vi "autonSample.vi"(0 "Auton Array":dbl[][](array[numeric]), 5 "LeftEncoder":dbl, 7 "RightEncoder":dbl, 11 "MeasuredHeading":dbl) -> (4 "Left Drive":dbl, 6 "Right Drive":dbl, 8 "Ramp ACT motor":dbl, 10 "Harvester":dbl, 13 "Shooter motor output":dbl, 14 "Turret Rotation":dbl, 15 "Convyeor":dbl)   [LabVIEW 2011]
uses:
  <vilib>/addons/Kinect/Skeleton Vertex Index.ctl
  Robot Global Data.vi
panel:
  out "Primitive ID":i16
  out "Tzero":i64
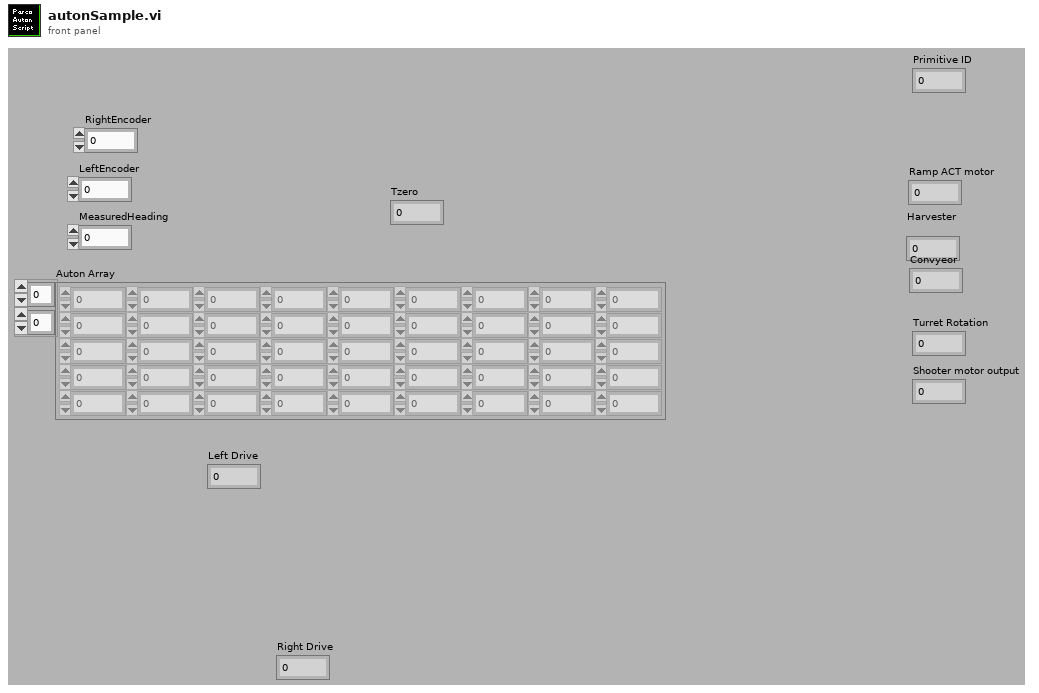
[diagram p1: front panel]
types:
  T1 = typedef "Skeleton Vertex Index.ctl" = i32
  T2 = cluster{"RightAxis":dbl, "LeftAxis":dbl, "RightHead":bool, "Left Head":bool, "Left Leg Out":bool, "Left Leg Forward":bool, "Left Leg Back":bool, "Right Leg Out":bool, "Right Leg Forward":bool, "Right Leg Back":bool}
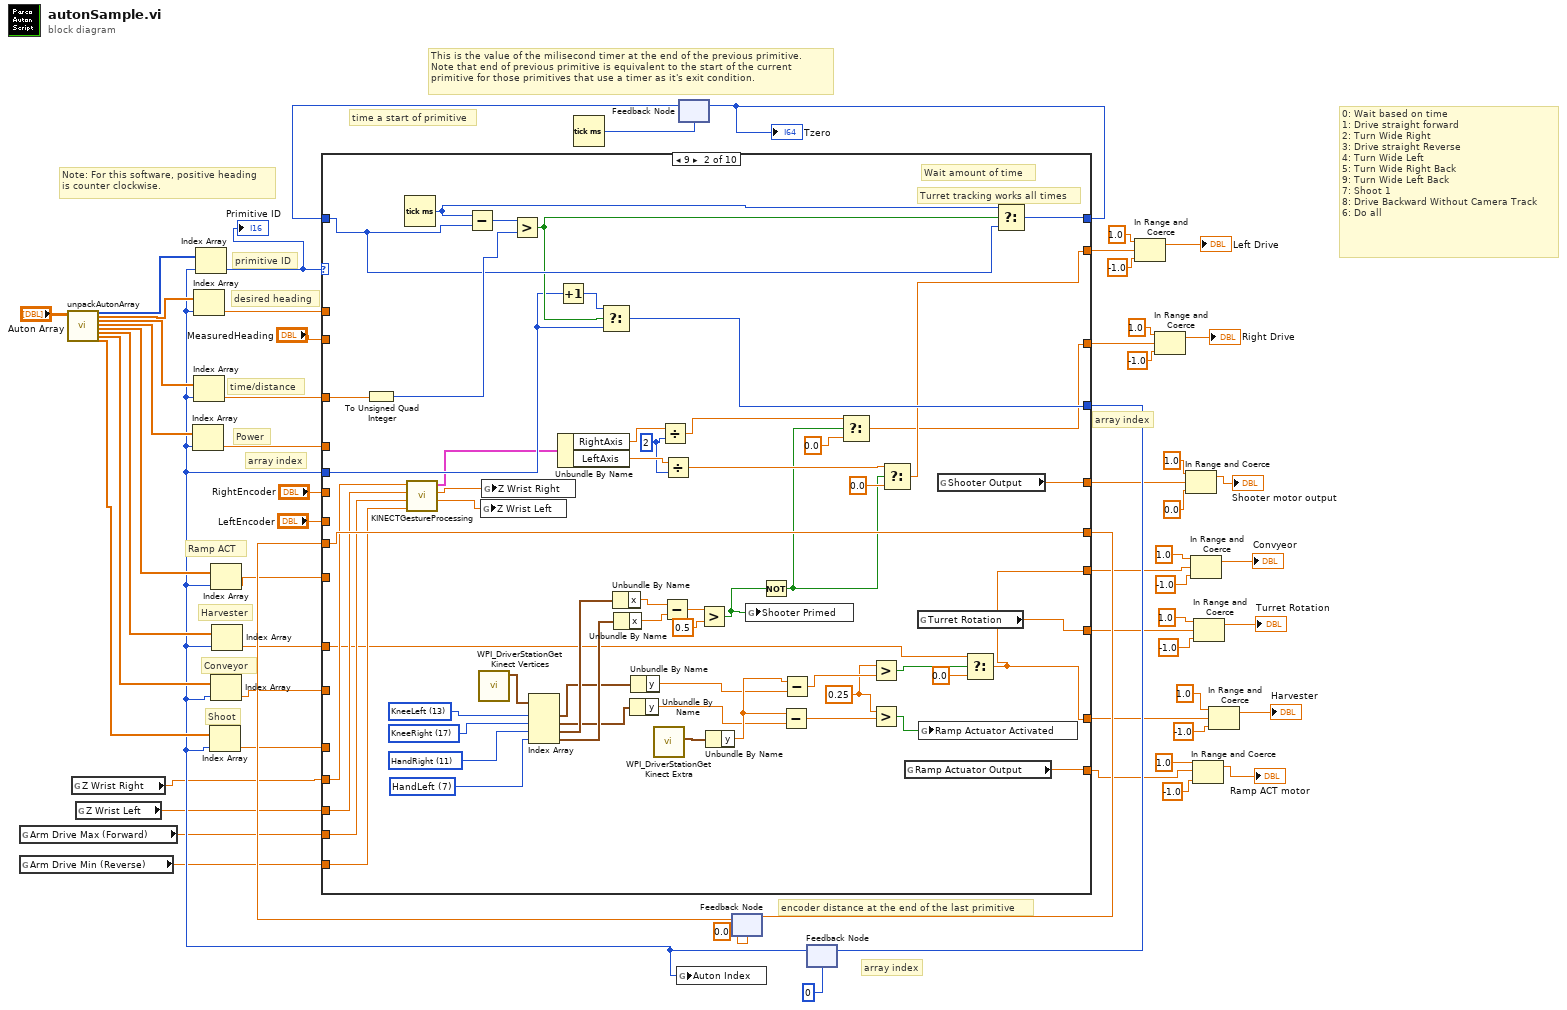
[diagram p0: block diagram]
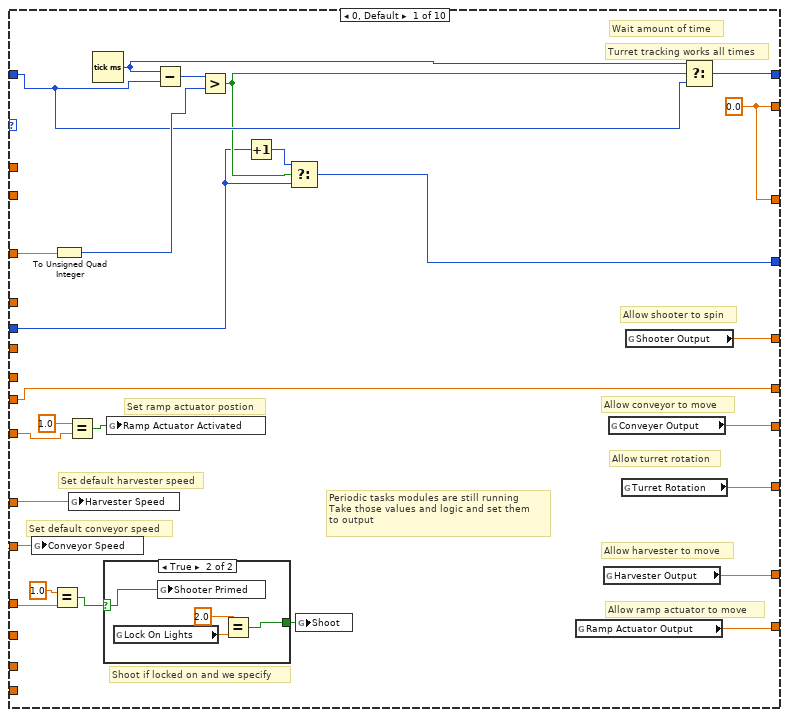
[diagram p2: hidden frame]
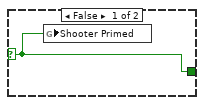
[diagram p3: hidden frame]
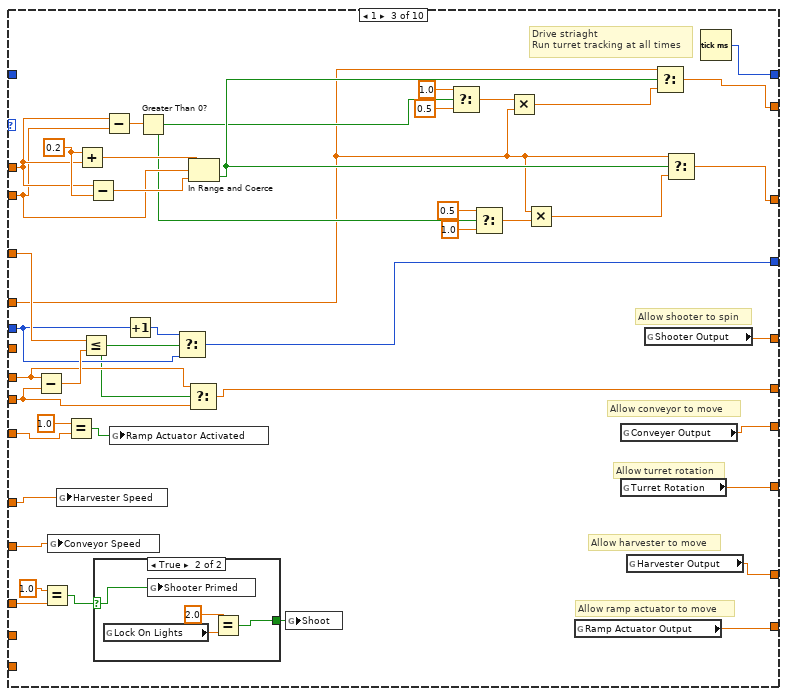
[diagram p4: hidden frame]
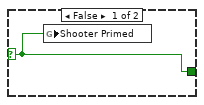
[diagram p5: hidden frame]
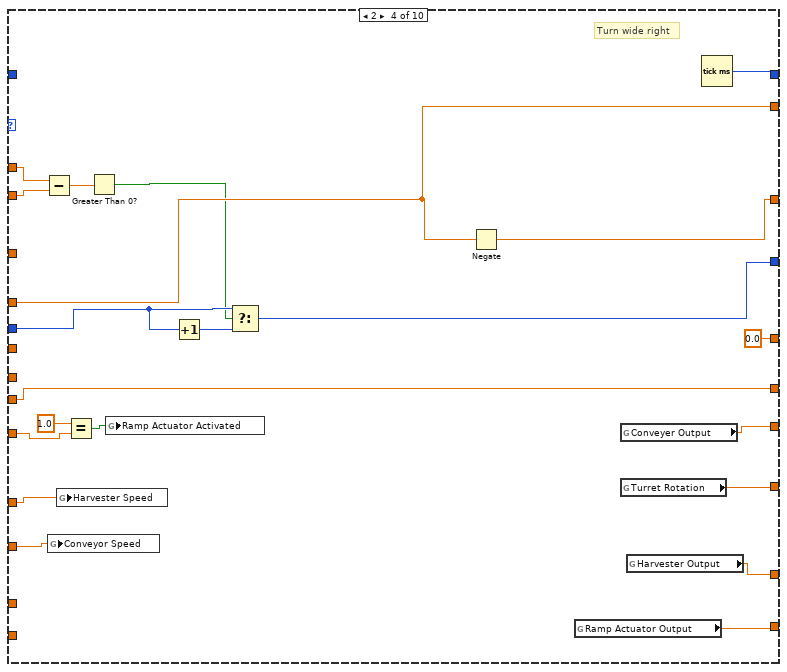
[diagram p6: hidden frame]
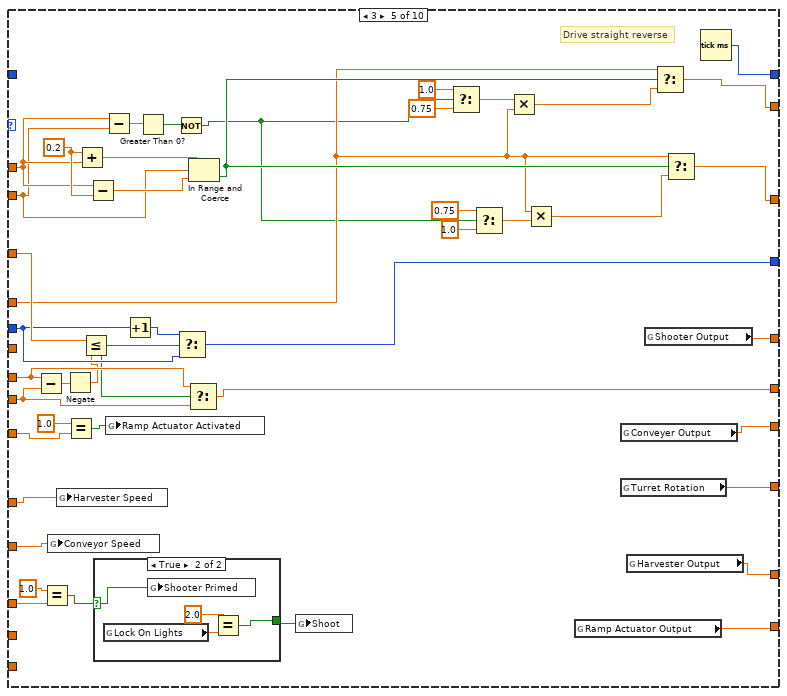
[diagram p7: hidden frame]
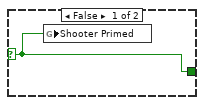
[diagram p8: hidden frame]
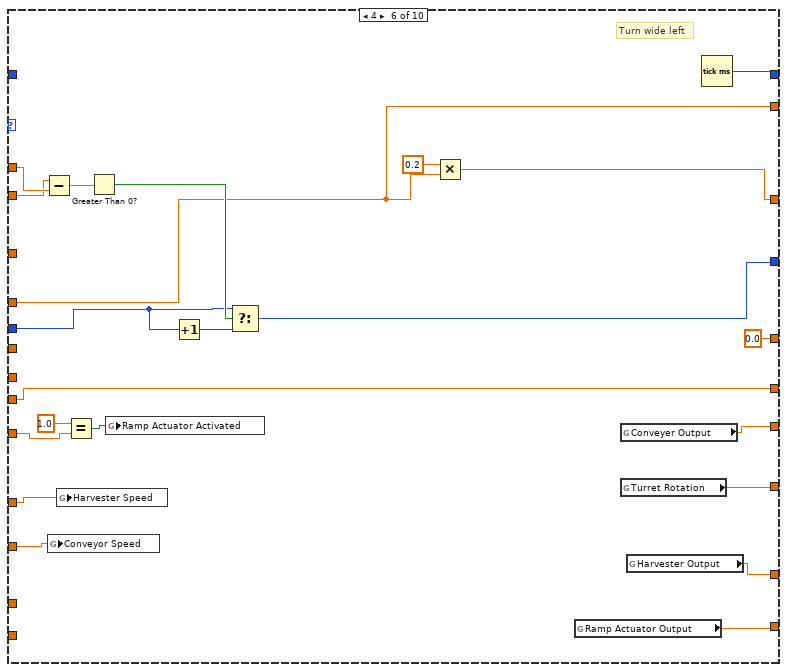
[diagram p9: hidden frame]
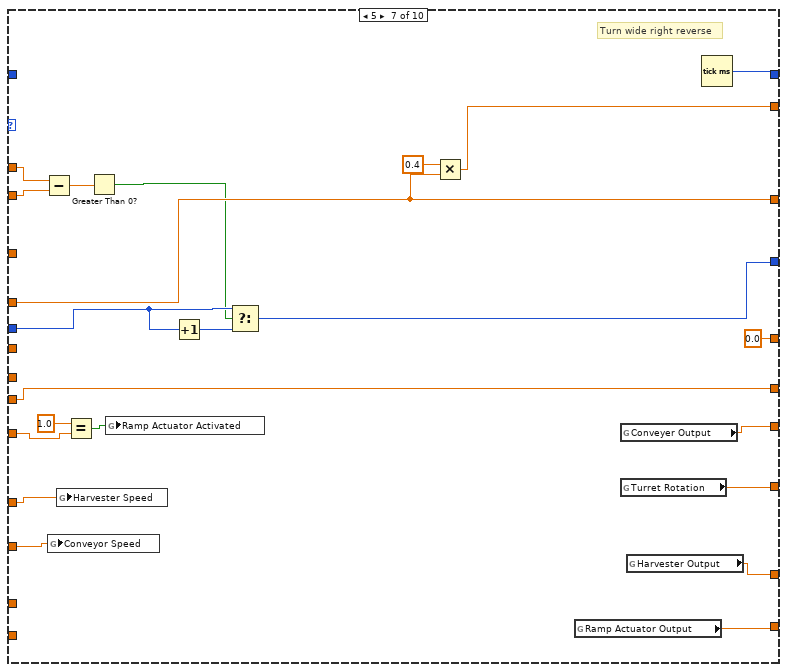
[diagram p10: hidden frame]
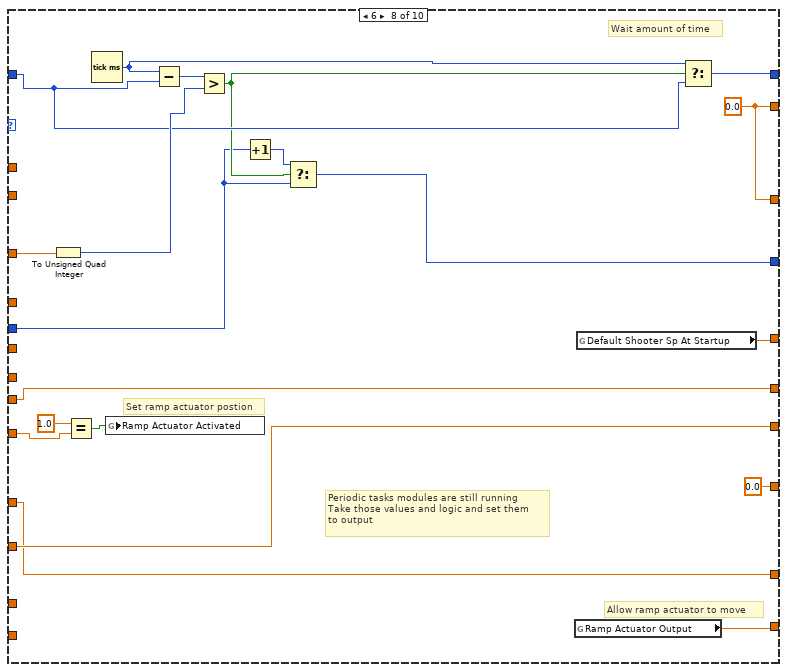
[diagram p11: hidden frame]
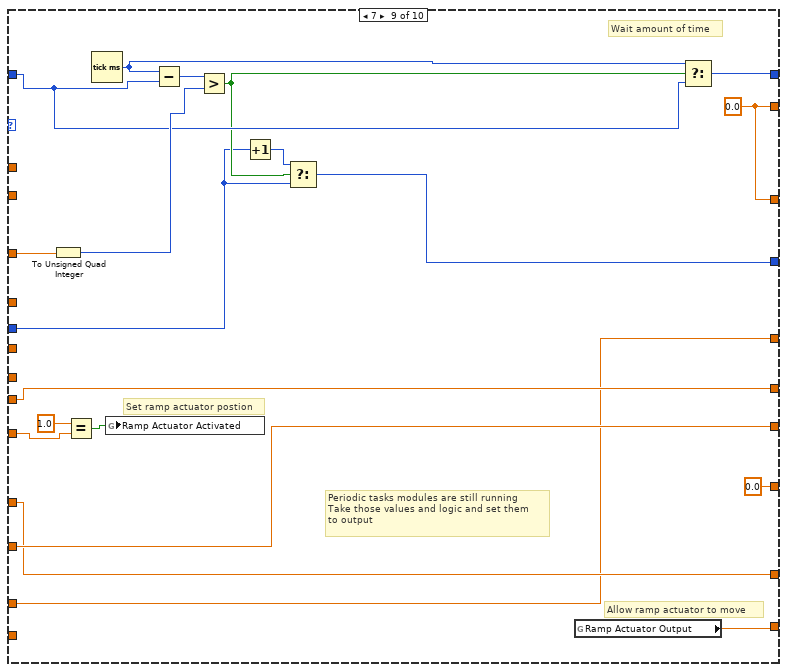
[diagram p12: hidden frame]
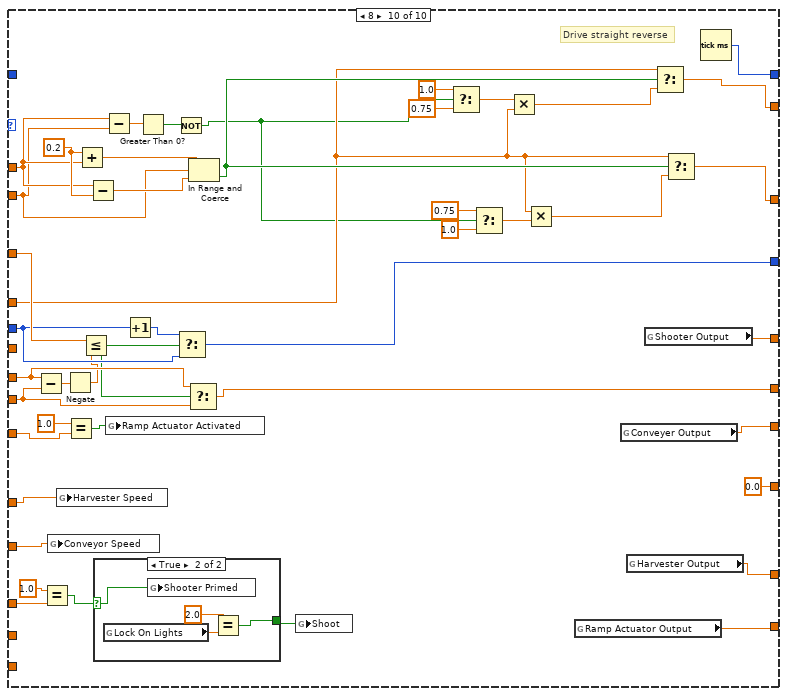
[diagram p13: hidden frame]
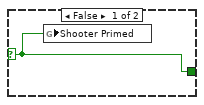
[diagram p14: hidden frame]
diagram:
  # "0: Wait based on time\n1: Drive straight forward\n2: Turn Wide Right\n3: Drive straight Reverse\n4: Turn Wide Left\n5: Turn Wide Right Back\n9: Turn Wide Left Back\n7: Shoot 1\n8: Drive Backward Without Camera Track\n6: Do all"
  # "Shoot"
  # "Conveyor"
  # "Harvester"
  # "Ramp ACT"
  # "encoder distance at the end of the last primitive"
  # "Note: For this software, positive heading\nis counter clockwise."
  # "time a start of primitive"
  # "array index"
  # "array index"
  # "This is the value of the milisecond timer at the end of the previous primitive.\nNote that end of previous primitive is equivalent to the start of the current\nprimitive for those primitives that use a timer as it's exit condition."
  # "Power"
  # "array index"
  # "desired heading"
  # "primitive ID"
  # "time/distance"
  n1 = global read "Robot Global Data.vi" "Arm Drive Max (Forward)"() -> (w2:dbl)
  n2 = global read "Robot Global Data.vi" "Arm Drive Min (Reverse)"() -> (w1:dbl)
  n3 = call "unpackAutonArray.vi"("all rows"="Auton Array") -> ("Primitive"=w60:i16[], "Desired Heading"=w20:dbl[], "Time/Distance"=w19:dbl[], "Power"=w18:dbl[], "Ramp Actuator"=w17:dbl[], "Harvester"=w16:dbl[], "Conveyor"=w15:dbl[], "Shoot"=w14:dbl[])  [unwired: 1 in, 18 out]
  n4 = global read "Robot Global Data.vi" "Z Wrist Right"() -> (w4:dbl)
  n5 = global read "Robot Global Data.vi" "Z Wrist Left"() -> (w3:dbl)
  n6 = Tick Count (ms)() -> (millisecond timer value=w55:u32)
  n7 = feedback #1(w55) -> (w59:u32)
  n8 = feedback #2(0.0 ("EncoderDistance")) -> (w43:dbl)
  n9 = feedback #3(0) -> (w12:i32)
  n10 = Index Array(array=w18, index=w12) -> (element=w57:dbl)
  n11 = Index Array(array=w20, index=w12) -> (element=w44:dbl)
  n12 = Index Array(array=w19, index=w12) -> (element=w58:dbl)
  n13 = Index Array(array=w60, index=w12) -> (element=w26:i16)
  "Primitive ID" <- w26
  n14 = Index Array(array=w14, index=w12) -> (element=w13:dbl)
  n15 = Index Array(array=w17, index=w12) -> (element=w25:dbl)
  n16 = Index Array(array=w15, index=w12) -> (element=w10:dbl)
  n17 = Index Array(array=w16, index=w12) -> (element=w11:dbl)
  n18 = case shown="9" w26 {
    tunnel: [w79 w141 w175 w201 w247 w274 w292 w324 w344 w382] -> w39
    tunnel: w12 -> [w80 w142 w177 w203 w249 w276 w294 w325 w345 w384]
    tunnel: [w87 w149 w153 w207 w226 w280 w301 w332 w352 w361] -> w45
    tunnel: w59 -> [w84 w146 _ _ _ _ _ w329 w349 _]
    tunnel: w58 -> [w73 w140 w178 _ w250 _ _ w319 w339 w385]
    tunnel: w44 -> [_ _ w166 w206 w238 w271 w300 _ _ w373]
    tunnel: [w78 w123 w152 w200 w225 w273 w296 w323 w343 w360] -> w53
    tunnel: [w78 w122 w151 w199 w224 w272 w298 w323 w343 w359] -> w46
    tunnel: w57 -> [_ _ w155 w200 w228 w273 w298 _ _ w363]
    tunnel: "LeftEncoder" -> [_ _ w172 _ w244 _ _ _ _ w379]
    tunnel: "MeasuredHeading" -> [_ _ w165 w205 w237 w270 w299 _ _ w372]
    tunnel: [w72 w139 w174 w209 w246 w282 w303 w318 w338 w381] -> w40
    tunnel: w43 -> [w72 w139 w173 w209 w245 w282 w303 w318 w338 w380]
    tunnel: [w62 w138 w180 0.0 ("Shooter Output") w251 0.0 ("Shooter Output") 0.0 ("Shooter Output") w313 w333 w386] -> w35
    tunnel: [w74 w95 w190 w215 w260 w287 w309 0.0 ("Turret Rotation") 0.0 ("Turret Rotation") 0.0 ("Turret Rotation")] -> w31
    tunnel: [w70 w96 w184 w211 w255 w284 w305 w315 w335 w390] -> w27
    tunnel: w25 -> [w67 _ w187 w214 w223 w269 w308 w317 w337 w358]
    tunnel: [w75 w94 w191 w216 w261 w288 w310 w320 w340 w395] -> w24
    tunnel: w13 -> [w63 _ w188 _ w258 _ _ _ w333 w393]
    tunnel: w11 -> [w68 w97 w186 w213 w257 w286 w307 w315 w335 w392]
    tunnel: w10 -> [w69 _ w185 w212 w256 w285 w306 w316 w336 w391]
    tunnel: [w71 w96 w183 w210 w254 w283 w304 w316 w336 w389] -> w6
    tunnel: "RightEncoder" -> [_ _ _ _ _ _ _ _ _ _]
    tunnel: w4 -> [_ w137 _ _ _ _ _ _ _ _]
    tunnel: w3 -> [_ w136 _ _ _ _ _ _ _ _]
    tunnel: w2 -> [_ w135 _ _ _ _ _ _ _ _]
    tunnel: w1 -> [_ w134 _ _ _ _ _ _ _ _]
    frame 0, Default {
      w78 = 0.0 ("Numeric")
      # "Periodic tasks modules are still running\nTake those values and logic and set them \nto output"
      # "Set ramp actuator postion"
      # "Set default harvester speed"
      # "Set default conveyor speed"
      # "Shoot if locked on and we specify"
      # "Allow ramp actuator to move"
      # "Allow harvester to move"
      # "Turret tracking works all times"
      # "Allow turret rotation"
      # "Allow conveyor to move"
      # "Allow shooter to spin"
      # "Wait amount of time"
      n19 = global write "Robot Global Data.vi" "Conveyor Speed"(w69) -> ()
      n20 = Equal?(x=1.0, y=w63) -> (x = y?=w65:bool)
      n21 = To Unsigned Quad Integer(1:w73) -> (0:w85:u64)
      n22 = Equal?(x=1.0, y=w67) -> (x = y?=w76:bool)
      n23 = global write "Robot Global Data.vi" "Harvester Speed"(w68) -> ()
      n24 = Tick Count (ms)() -> (millisecond timer value=w83:u32)
      n25 = case shown="True" w65 {
        selector: w65 -> [w88 w92]
        tunnel: [w88 w89] -> w64
        frame False {
          n26 = global write "Robot Global Data.vi" "Shooter Primed"(w88) -> ()
        }
        frame True {
          n27 = global read "Robot Global Data.vi" "Lock On Lights"() -> (w90:dbl)
          n28 = global write "Robot Global Data.vi" "Shooter Primed"(w92) -> ()
          n29 = Equal?(x=2.0, y=w90) -> (x = y?=w89:bool)
        }
      }
      n30 = global write "Robot Global Data.vi" "Ramp Actuator Activated"(w76) -> ()
      n31 = Subtract(x=w83, y=w84) -> (x-y=w86:u32)
      n32 = Greater?(x=w86, y=w85) -> (0:w82:bool)
      n33 = Increment(x=w80) -> (x+1=w81:i32)
      n34 = Select(t=w81, s=w82, f=w80) -> (s? t:f=w79:i32)
      n35 = global write "Robot Global Data.vi" "Shoot"(w64) -> ()
      n36 = global read "Robot Global Data.vi" "Ramp Actuator Output"() -> (w75:dbl)
      n37 = global read "Robot Global Data.vi" "Harvester Output"() -> (w70:dbl)
      n38 = global read "Robot Global Data.vi" "Conveyer Output"() -> (w71:dbl)
      n39 = global read "Robot Global Data.vi" "Turret Rotation"() -> (w74:dbl)
      n40 = global read "Robot Global Data.vi" "Shooter Output"() -> (w62:dbl)
      n41 = Select(t=w83, s=w82, f=w84) -> (s? t:f=w87:u32)
    }
    frame 9 {
      w100 = 0.25
      w117 = T1 7 items=["HipCenter", "Spine", "ShoulderCenter", "Head", "ShoulderLeft", "ElbowLeft", "WristLeft", "HandLeft", "ShoulderRight", "ElbowRight", "WristRight", "HandRight", "HipLeft", "KneeLeft", "AnkleLeft", "FootLeft", "HipRight", "KneeRight", "AnkleRight", "FootRight"] ("Skeleton Joints")
      w118 = T1 11 items=["HipCenter", "Spine", "ShoulderCenter", "Head", "ShoulderLeft", "ElbowLeft", "WristLeft", "HandLeft", "ShoulderRight", "ElbowRight", "WristRight", "HandRight", "HipLeft", "KneeLeft", "AnkleLeft", "FootLeft", "HipRight", "KneeRight", "AnkleRight", "FootRight"] ("Skeleton Joints")
      w119 = T1 17 items=["HipCenter", "Spine", "ShoulderCenter", "Head", "ShoulderLeft", "ElbowLeft", "WristLeft", "HandLeft", "ShoulderRight", "ElbowRight", "WristRight", "HandRight", "HipLeft", "KneeLeft", "AnkleLeft", "FootLeft", "HipRight", "KneeRight", "AnkleRight", "FootRight"] ("Skeleton Joints")
      w120 = T1 13 items=["HipCenter", "Spine", "ShoulderCenter", "Head", "ShoulderLeft", "ElbowLeft", "WristLeft", "HandLeft", "ShoulderRight", "ElbowRight", "WristRight", "HandRight", "HipLeft", "KneeLeft", "AnkleLeft", "FootLeft", "HipRight", "KneeRight", "AnkleRight", "FootRight"] ("Skeleton Joints")
      w128 = 2
      # "Turret tracking works all times"
      # "Wait amount of time"
      n42 = To Unsigned Quad Integer(1:w140) -> (0:w147:u64)
      n43 = Tick Count (ms)() -> (millisecond timer value=w145:u32)
      n44 = call "KINECTGestureProcessing.vi"("Z Wrist Right in"=w137, "Z Wrist Left in"=w136, "Arm Drive in Max (Forward)"=w135, "Arm Drive in Min (Reverse)"=w134) -> ("Joystick Data"=w131:T2, "Z Wrist Right out"=w133:dbl, "Z Wrist Left out"=w132:dbl)  [unwired: 2 in]
      n45 = Subtract(x=w145, y=w146) -> (x-y=w148:u32)
      n46 = call <vilib>:"WPI_DriverStationGet Kinect Vertices.vi"() -> ("Skeleton Vertices"=w121:cluster{"x":sgl, "y":sgl, "z":sgl}[])  [unwired: 10 in, 1 out]
      n47 = global write "Robot Global Data.vi" "Z Wrist Left"(w132) -> ()
      n48 = global write "Robot Global Data.vi" "Z Wrist Right"(w133) -> ()
      n49 = Greater?(x=w148, y=w147) -> (0:w144:bool)
      n50 = Index Array(array=w121, index #1=w120, index #2=w119, index #3=w118, index #4=w117) -> (element #1=w114:cluster{"x":sgl, "y":sgl, "z":sgl}, element #2=w113:cluster{"x":sgl, "y":sgl, "z":sgl}, element #3=w116:cluster{"x":sgl, "y":sgl, "z":sgl}, element #4=w115:cluster{"x":sgl, "y":sgl, "z":sgl})
      n51 = Increment(x=w142) -> (x+1=w143:i32)
      n52 = Unbundle By Name(w131) -> ("RightAxis"=w130:dbl, "LeftAxis"=w129:dbl)
      n53 = Select(t=w143, s=w144, f=w142) -> (s? t:f=w141:i32)
      n54 = Unbundle By Name(w116) -> ("x"=w112:sgl)
      n55 = Unbundle By Name(w115) -> ("x"=w111:sgl)
      n56 = Unbundle By Name(w113) -> ("y"=w104:sgl)
      n57 = Unbundle By Name(w114) -> ("y"=w103:sgl)
      n58 = call <vilib>:"WPI_DriverStationGet Kinect Extra.vi"() -> ("Overall Position"=w106:cluster{"x":sgl, "y":sgl, "z":sgl})  [unwired: 7 in, 4 out]
      n59 = Divide(x=w130, y=w128) -> (x/y=w127:dbl)
      n60 = Subtract(x=w112, y=w111) -> (x-y=w110:sgl)
      n61 = Divide(x=w129, y=w128) -> (x/y=w126:dbl)
      n62 = Greater?(x=w110, y=sgl 0.5) -> (0:w108:bool)
      n63 = Unbundle By Name(w106) -> ("y"=w105:sgl)
      n64 = global write "Robot Global Data.vi" "Shooter Primed"(w108) -> ()
      n65 = Not(x=w108) -> (.not. x?=w107:bool)
      n66 = Subtract(x=w105, y=w104) -> (x-y=w102:sgl)
      n67 = Subtract(x=w105, y=w103) -> (x-y=w101:sgl)
      n68 = Select(t=w127, s=w107, f=0.0) -> (s? t:f=w122:dbl)
      n69 = Greater?(x=w100, y=w101) -> (0:w99:bool)
      n70 = Greater?(x=w100, y=w102) -> (0:w93:bool)
      n71 = Select(t=w126, s=w107, f=0.0) -> (s? t:f=w123:dbl)
      n72 = global read "Robot Global Data.vi" "Ramp Actuator Output"() -> (w94:dbl)
      n73 = global read "Robot Global Data.vi" "Turret Rotation"() -> (w95:dbl)
      n74 = global write "Robot Global Data.vi" "Ramp Actuator Activated"(w93) -> ()
      n75 = global read "Robot Global Data.vi" "Shooter Output"() -> (w138:dbl)
      n76 = Select(t=w97, s=w99, f=0.0) -> (s? t:f=w96:dbl)
      n77 = Select(t=w145, s=w144, f=w146) -> (s? t:f=w149:u32)
    }
    frame 1 {
      w170 = 0.2 ("x")
      # "Allow ramp actuator to move"
      # "Allow harvester to move"
      # "Allow turret rotation"
      # "Allow conveyor to move"
      # "Allow shooter to spin"
      # "Drive striaght\nRun turret tracking at all times"
      n78 = Subtract(x=w172, y=w173) -> (x-y=w179:dbl)
      n79 = Equal?(x=1.0, y=w188) -> (x = y?=w182:bool)
      n80 = global write "Robot Global Data.vi" "Conveyor Speed"(w185) -> ()
      n81 = global write "Robot Global Data.vi" "Harvester Speed"(w186) -> ()
      n82 = Equal?(x=1.0, y=w187) -> (x = y?=w150:bool)
      n83 = Add(x=w170, y=w166) -> (x+y=w168:dbl)
      n84 = Less Or Equal?(x=w178, y=w179) -> (x <= y?=w171:bool)
      n85 = Subtract(x=w166, y=w170) -> (x-y=w169:dbl)
      n86 = case shown="True" w182 {
        selector: w182 -> [w193 w197]
        tunnel: [w193 w194] -> w181
        frame False {
          n87 = global write "Robot Global Data.vi" "Shooter Primed"(w193) -> ()
        }
        frame True {
          n88 = global read "Robot Global Data.vi" "Lock On Lights"() -> (w195:dbl)
          n89 = global write "Robot Global Data.vi" "Shooter Primed"(w197) -> ()
          n90 = Equal?(x=2.0, y=w195) -> (x = y?=w194:bool)
        }
      }
      n91 = Subtract(x=w166, y=w165) -> (x-y=w164:dbl)
      n92 = global write "Robot Global Data.vi" "Ramp Actuator Activated"(w150) -> ()
      n93 = Increment(x=w177) -> (x+1=w176:i32)
      n94 = Greater Than 0?(x=w164) -> (x > 0?=w163:bool)
      n95 = Select(t=w176, s=w171, f=w177) -> (s? t:f=w175:i32)
      n96 = Select(t=w172, s=w171, f=w173) -> (s? t:f=w174:dbl)
      n97 = In Range and Coerce(upper limit=w168, x=w165, lower limit=w169) -> (In Range?=w167:bool)  [unwired: 1 out]
      n98 = global write "Robot Global Data.vi" "Shoot"(w181) -> ()
      n99 = Select(t=1.0, s=w163, f=0.5) -> (s? t:f=w156:dbl)
      n100 = Select(t=0.5, s=w163, f=1.0) -> (s? t:f=w158:dbl)
      n101 = Multiply(x=w156, y=w155) -> (x*y=w154:dbl)
      n102 = Multiply(x=w155, y=w158) -> (x*y=w157:dbl)
      n103 = global read "Robot Global Data.vi" "Ramp Actuator Output"() -> (w191:dbl)
      n104 = global read "Robot Global Data.vi" "Conveyer Output"() -> (w183:dbl)
      n105 = global read "Robot Global Data.vi" "Turret Rotation"() -> (w190:dbl)
      n106 = global read "Robot Global Data.vi" "Harvester Output"() -> (w184:dbl)
      n107 = global read "Robot Global Data.vi" "Shooter Output"() -> (w180:dbl)
      n108 = Select(t=w155, s=w167, f=w154) -> (s? t:f=w152:dbl)
      n109 = Select(t=w155, s=w167, f=w157) -> (s? t:f=w151:dbl)
      n110 = Tick Count (ms)() -> (millisecond timer value=w153:u32)
    }
    frame 2 {
      # "Turn wide right"
      n111 = Subtract(x=w206, y=w205) -> (x-y=w204:dbl)
      n112 = global write "Robot Global Data.vi" "Conveyor Speed"(w212) -> ()
      n113 = global write "Robot Global Data.vi" "Harvester Speed"(w213) -> ()
      n114 = Equal?(x=1.0, y=w214) -> (x = y?=w217:bool)
      n115 = Greater Than 0?(x=w204) -> (x > 0?=w198:bool)
      n116 = global write "Robot Global Data.vi" "Ramp Actuator Activated"(w217) -> ()
      n117 = Increment(x=w203) -> (x+1=w202:i32)
      n118 = Select(t=w203, s=w198, f=w202) -> (s? t:f=w201:i32)
      n119 = Negate(x=w200) -> (-x=w199:dbl)
      n120 = global read "Robot Global Data.vi" "Ramp Actuator Output"() -> (w216:dbl)
      n121 = global read "Robot Global Data.vi" "Conveyer Output"() -> (w210:dbl)
      n122 = global read "Robot Global Data.vi" "Turret Rotation"() -> (w215:dbl)
      n123 = global read "Robot Global Data.vi" "Harvester Output"() -> (w211:dbl)
      n124 = Tick Count (ms)() -> (millisecond timer value=w207:u32)
    }
    frame 3 {
      w242 = 0.2 ("x")
      # "Drive straight reverse"
      n125 = Subtract(x=w244, y=w245) -> (x-y=w222:dbl)
      n126 = Equal?(x=1.0, y=w258) -> (x = y?=w253:bool)
      n127 = global write "Robot Global Data.vi" "Conveyor Speed"(w256) -> ()
      n128 = global write "Robot Global Data.vi" "Harvester Speed"(w257) -> ()
      n129 = Negate(x=w222) -> (-x=w221:dbl)
      n130 = Equal?(x=1.0, y=w223) -> (x = y?=w262:bool)
      n131 = Add(x=w242, y=w238) -> (x+y=w240:dbl)
      n132 = Less Or Equal?(x=w250, y=w221) -> (x <= y?=w243:bool)
      n133 = Subtract(x=w238, y=w242) -> (x-y=w241:dbl)
      n134 = case shown="True" w253 {
        selector: w253 -> [w264 w268]
        tunnel: [w264 w265] -> w252
        frame False {
          n135 = global write "Robot Global Data.vi" "Shooter Primed"(w264) -> ()
        }
        frame True {
          n136 = global read "Robot Global Data.vi" "Lock On Lights"() -> (w266:dbl)
          n137 = global write "Robot Global Data.vi" "Shooter Primed"(w268) -> ()
          n138 = Equal?(x=2.0, y=w266) -> (x = y?=w265:bool)
        }
      }
      n139 = Subtract(x=w238, y=w237) -> (x-y=w236:dbl)
      n140 = global write "Robot Global Data.vi" "Ramp Actuator Activated"(w262) -> ()
      n141 = Increment(x=w249) -> (x+1=w248:i32)
      n142 = Greater Than 0?(x=w236) -> (x > 0?=w220:bool)
      n143 = Not(x=w220) -> (.not. x?=w219:bool)
      n144 = Select(t=w248, s=w243, f=w249) -> (s? t:f=w247:i32)
      n145 = Select(t=w244, s=w243, f=w245) -> (s? t:f=w246:dbl)
      n146 = In Range and Coerce(upper limit=w240, x=w237, lower limit=w241) -> (In Range?=w239:bool)  [unwired: 1 out]
      n147 = global write "Robot Global Data.vi" "Shoot"(w252) -> ()
      n148 = Select(t=1.0, s=w219, f=0.75) -> (s? t:f=w229:dbl)
      n149 = Select(t=0.75, s=w219, f=1.0) -> (s? t:f=w231:dbl)
      n150 = Multiply(x=w229, y=w228) -> (x*y=w227:dbl)
      n151 = Multiply(x=w228, y=w231) -> (x*y=w230:dbl)
      n152 = global read "Robot Global Data.vi" "Ramp Actuator Output"() -> (w261:dbl)
      n153 = global read "Robot Global Data.vi" "Conveyer Output"() -> (w254:dbl)
      n154 = global read "Robot Global Data.vi" "Turret Rotation"() -> (w260:dbl)
      n155 = global read "Robot Global Data.vi" "Harvester Output"() -> (w255:dbl)
      n156 = global read "Robot Global Data.vi" "Shooter Output"() -> (w251:dbl)
      n157 = Select(t=w228, s=w239, f=w227) -> (s? t:f=w225:dbl)
      n158 = Select(t=w228, s=w239, f=w230) -> (s? t:f=w224:dbl)
      n159 = Tick Count (ms)() -> (millisecond timer value=w226:u32)
    }
    frame 4 {
      # "Turn wide left"
      n160 = Subtract(x=w270, y=w271) -> (x-y=w278:dbl)
      n161 = global write "Robot Global Data.vi" "Conveyor Speed"(w285) -> ()
      n162 = global write "Robot Global Data.vi" "Harvester Speed"(w286) -> ()
      n163 = Equal?(x=1.0, y=w269) -> (x = y?=w289:bool)
      n164 = Greater Than 0?(x=w278) -> (x > 0?=w277:bool)
      n165 = global write "Robot Global Data.vi" "Ramp Actuator Activated"(w289) -> ()
      n166 = Increment(x=w276) -> (x+1=w275:i32)
      n167 = Select(t=w276, s=w277, f=w275) -> (s? t:f=w274:i32)
      n168 = Multiply(x=0.2, y=w273) -> (x*y=w272:dbl)
      n169 = global read "Robot Global Data.vi" "Ramp Actuator Output"() -> (w288:dbl)
      n170 = global read "Robot Global Data.vi" "Conveyer Output"() -> (w283:dbl)
      n171 = global read "Robot Global Data.vi" "Turret Rotation"() -> (w287:dbl)
      n172 = global read "Robot Global Data.vi" "Harvester Output"() -> (w284:dbl)
      n173 = Tick Count (ms)() -> (millisecond timer value=w280:u32)
    }
    frame 5 {
      # "Turn wide right reverse"
      n174 = Subtract(x=w300, y=w299) -> (x-y=w295:dbl)
      n175 = global write "Robot Global Data.vi" "Conveyor Speed"(w306) -> ()
      n176 = global write "Robot Global Data.vi" "Harvester Speed"(w307) -> ()
      n177 = Equal?(x=1.0, y=w308) -> (x = y?=w311:bool)
      n178 = Greater Than 0?(x=w295) -> (x > 0?=w291:bool)
      n179 = global write "Robot Global Data.vi" "Ramp Actuator Activated"(w311) -> ()
      n180 = Increment(x=w294) -> (x+1=w293:i32)
      n181 = Select(t=w294, s=w291, f=w293) -> (s? t:f=w292:i32)
      n182 = Multiply(x=0.4, y=w298) -> (x*y=w296:dbl)
      n183 = global read "Robot Global Data.vi" "Ramp Actuator Output"() -> (w310:dbl)
      n184 = global read "Robot Global Data.vi" "Conveyer Output"() -> (w304:dbl)
      n185 = global read "Robot Global Data.vi" "Turret Rotation"() -> (w309:dbl)
      n186 = global read "Robot Global Data.vi" "Harvester Output"() -> (w305:dbl)
      n187 = Tick Count (ms)() -> (millisecond timer value=w301:u32)
    }
    frame 6 {
      w323 = 0.0 ("Numeric")
      # "Periodic tasks modules are still running\nTake those values and logic and set them \nto output"
      # "Set ramp actuator postion"
      # "Allow ramp actuator to move"
      # "Wait amount of time"
      n188 = To Unsigned Quad Integer(1:w319) -> (0:w330:u64)
      n189 = Equal?(x=1.0, y=w317) -> (x = y?=w321:bool)
      n190 = Tick Count (ms)() -> (millisecond timer value=w328:u32)
      n191 = global write "Robot Global Data.vi" "Ramp Actuator Activated"(w321) -> ()
      n192 = Subtract(x=w328, y=w329) -> (x-y=w331:u32)
      n193 = Greater?(x=w331, y=w330) -> (0:w327:bool)
      n194 = Increment(x=w325) -> (x+1=w326:i32)
      n195 = Select(t=w326, s=w327, f=w325) -> (s? t:f=w324:i32)
      n196 = global read "Robot Global Data.vi" "Ramp Actuator Output"() -> (w320:dbl)
      n197 = global read "Robot Global Data.vi" "Default Shooter Sp At Startup"() -> (w313:dbl)
      n198 = Select(t=w328, s=w327, f=w329) -> (s? t:f=w332:u32)
    }
    frame 7 {
      w343 = 0.0 ("Numeric")
      # "Periodic tasks modules are still running\nTake those values and logic and set them \nto output"
      # "Set ramp actuator postion"
      # "Allow ramp actuator to move"
      # "Wait amount of time"
      n199 = To Unsigned Quad Integer(1:w339) -> (0:w350:u64)
      n200 = Equal?(x=1.0, y=w337) -> (x = y?=w341:bool)
      n201 = Tick Count (ms)() -> (millisecond timer value=w348:u32)
      n202 = global write "Robot Global Data.vi" "Ramp Actuator Activated"(w341) -> ()
      n203 = Subtract(x=w348, y=w349) -> (x-y=w351:u32)
      n204 = Greater?(x=w351, y=w350) -> (0:w347:bool)
      n205 = Increment(x=w345) -> (x+1=w346:i32)
      n206 = Select(t=w346, s=w347, f=w345) -> (s? t:f=w344:i32)
      n207 = global read "Robot Global Data.vi" "Ramp Actuator Output"() -> (w340:dbl)
      n208 = Select(t=w348, s=w347, f=w349) -> (s? t:f=w352:u32)
    }
    frame 8 {
      w377 = 0.2 ("x")
      # "Drive straight reverse"
      n209 = Subtract(x=w379, y=w380) -> (x-y=w357:dbl)
      n210 = Equal?(x=1.0, y=w393) -> (x = y?=w388:bool)
      n211 = global write "Robot Global Data.vi" "Conveyor Speed"(w391) -> ()
      n212 = global write "Robot Global Data.vi" "Harvester Speed"(w392) -> ()
      n213 = Negate(x=w357) -> (-x=w356:dbl)
      n214 = Equal?(x=1.0, y=w358) -> (x = y?=w396:bool)
      n215 = Add(x=w377, y=w373) -> (x+y=w375:dbl)
      n216 = Less Or Equal?(x=w385, y=w356) -> (x <= y?=w378:bool)
      n217 = Subtract(x=w373, y=w377) -> (x-y=w376:dbl)
      n218 = case shown="True" w388 {
        selector: w388 -> [w398 w402]
        tunnel: [w398 w399] -> w387
        frame False {
          n219 = global write "Robot Global Data.vi" "Shooter Primed"(w398) -> ()
        }
        frame True {
          n220 = global read "Robot Global Data.vi" "Lock On Lights"() -> (w400:dbl)
          n221 = global write "Robot Global Data.vi" "Shooter Primed"(w402) -> ()
          n222 = Equal?(x=2.0, y=w400) -> (x = y?=w399:bool)
        }
      }
      n223 = Subtract(x=w373, y=w372) -> (x-y=w371:dbl)
      n224 = global write "Robot Global Data.vi" "Ramp Actuator Activated"(w396) -> ()
      n225 = Increment(x=w384) -> (x+1=w383:i32)
      n226 = Greater Than 0?(x=w371) -> (x > 0?=w355:bool)
      n227 = Not(x=w355) -> (.not. x?=w354:bool)
      n228 = Select(t=w383, s=w378, f=w384) -> (s? t:f=w382:i32)
      n229 = Select(t=w379, s=w378, f=w380) -> (s? t:f=w381:dbl)
      n230 = In Range and Coerce(upper limit=w375, x=w372, lower limit=w376) -> (In Range?=w374:bool)  [unwired: 1 out]
      n231 = global write "Robot Global Data.vi" "Shoot"(w387) -> ()
      n232 = Select(t=1.0, s=w354, f=0.75) -> (s? t:f=w364:dbl)
      n233 = Select(t=0.75, s=w354, f=1.0) -> (s? t:f=w366:dbl)
      n234 = Multiply(x=w364, y=w363) -> (x*y=w362:dbl)
      n235 = Multiply(x=w363, y=w366) -> (x*y=w365:dbl)
      n236 = global read "Robot Global Data.vi" "Ramp Actuator Output"() -> (w395:dbl)
      n237 = global read "Robot Global Data.vi" "Conveyer Output"() -> (w389:dbl)
      n238 = global read "Robot Global Data.vi" "Harvester Output"() -> (w390:dbl)
      n239 = global read "Robot Global Data.vi" "Shooter Output"() -> (w386:dbl)
      n240 = Select(t=w363, s=w374, f=w362) -> (s? t:f=w360:dbl)
      n241 = Select(t=w363, s=w374, f=w365) -> (s? t:f=w359:dbl)
      n242 = Tick Count (ms)() -> (millisecond timer value=w361:u32)
    }
  }
  "Tzero" <- w45
  n243 = global write "Robot Global Data.vi" "Auton Index"(w12) -> ()
  n244 = feedback-in #1(w45) -> ()
  n245 = feedback-in #2(w40) -> ()
  n246 = feedback-in #3(w39) -> ()
  n247 = In Range and Coerce(upper limit=1.0, x=w53, lower limit=-1.0) -> (coerced(x)=→"Left Drive":dbl)  [unwired: 1 out]
  n248 = In Range and Coerce(upper limit=1.0, x=w46, lower limit=-1.0) -> (coerced(x)=→"Right Drive":dbl)  [unwired: 1 out]
  n249 = In Range and Coerce(upper limit=1.0, x=w35, lower limit=0.0) -> (coerced(x)=→"Shooter motor output":dbl)  [unwired: 1 out]
  n250 = In Range and Coerce(upper limit=1.0, x=w6, lower limit=-1.0) -> (coerced(x)=→"Convyeor":dbl)  [unwired: 1 out]
  n251 = In Range and Coerce(upper limit=1.0, x=w24, lower limit=-1.0) -> (coerced(x)=→"Ramp ACT motor":dbl)  [unwired: 1 out]
  n252 = In Range and Coerce(upper limit=1.0, x=w31, lower limit=-1.0) -> (coerced(x)=→"Turret Rotation":dbl)  [unwired: 1 out]
  n253 = In Range and Coerce(upper limit=1.0, x=w27, lower limit=-1.0) -> (coerced(x)=→"Harvester":dbl)  [unwired: 1 out]
